vi "系列号查询.vi"() -> ()   [LabVIEW 2016, in "斯坦道多参数.lvlib"]
panel:
  in  "传感器系列号":T1
  in  "布尔":bool
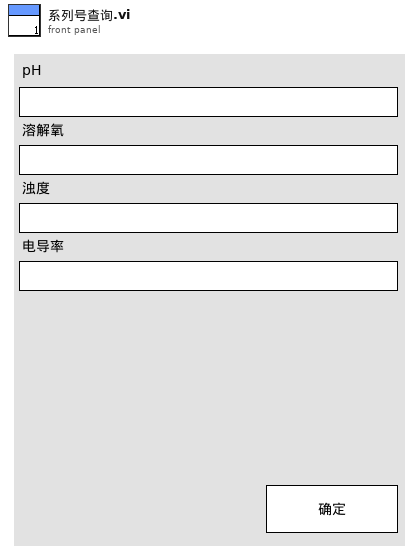
[diagram p1: front panel]
types:
  T1 = cluster{"pH":string, "溶解氧":string, "浊度":string, "电导率":string, "ORP":string, "叶绿素a":string, "藻密度":string}
  T2 = cluster{"pH探头选择":u16, "DO探头选择":u16, "电导率探头选择":u16, "浊度探头选择":u16, "叶绿素a探头选择":u16, "蓝绿藻探头选择":u16, "orp探头选择":u16, "COD探头选择":u16, "DO2探头选择":u16}
  T3 = enum16{"null", "pH", "DO", "浊度", "电导率", "叶绿素a", "DO2"}
  T4 = cluster{"电极状态标志":u16, "电极型号标志":u16, "电导率测量值":sgl, "温度测量值":sgl, "电导率信号值":sgl, "温度信号值":sgl, "温度补偿系数":sgl, "电导率偏移修正值":sgl, "温度偏移修正值":sgl, "手动温度补偿值":sgl, "电导率电极零点":sgl, "电导率电极斜率":sgl, "命令滤波设定":u16, "温度模式":enum16{"ATC", "MTC"}, "生产批次":u16, "电极序号":u16, "串口地址":u16, "串口波特率":enum16{"9600", "19200", "115200"}, "串口校验位":enum16{"NONE", "ODD", "EVEN"}, "串口停止位":enum16{"1bit", "2bit"}, "第一点标准值":sgl, "第二点标准值":sgl}
  T5 = cluster{"报警码":u16, "电导率数据（uS/cm）":sgl, "0x0003 NC":sgl, "温度数据":sgl, "电导率原始信号电阻":sgl, "当前量程":u16, "温度补偿系数":sgl, "0X0009_NC":string, "产品名称":string, "序列号":string, "硬件版本":string, "软件版本":string, "通讯地址":u16, "波特率":u16, "设备类型":u16, "0X0026_NC":string, "第一点原始数据":sgl, "第一点校准数据":sgl, "0X0035_NC":sgl, "0X0037_NC":sgl, "探头校准命令":u16, "温度校准参数":sgl, "温度校准命令":u16}
  T6 = cluster{"报警码":u16, "叶绿素a":sgl, "温度数据":sgl, "原始光强数值":u16, "量程":u16, "平均次数":u16, "清扫模式":u16, "清扫次数":u16, "清扫间隔分钟":u16, "0X000B_NC":string, "产品名称":string, "序列号":string, "硬件版本":string, "软件版本":string, "通讯地址":u16, "波特率":u16, "设备类型":u16, "0X0026_NC":string, "校准量程":u16, "第一点原始光强":u16, "第一点校准数据":sgl, "第二点原始光强":u16, "第二点校准数据":sgl, "第三点原始光强":u16, "第三点校准数据":sgl, "探头校准命令":u16, "温度校准参数":sgl, "温度校准命令":u16}
  T7 = cluster{"电极状态标志":u16, "电极型号标志":u16, "酸碱度测量值":sgl, "温度测量值":sgl, "酸碱度信号值":sgl, "温度信号值":sgl, "酸碱度偏移修正值":sgl, "温度偏移修正值":sgl, "手动温度补偿值":sgl, "酸碱度电极零点":sgl, "酸碱度电极斜率":sgl, "第1点标准值记录":sgl, "第1点信号值记录":sgl, "第1点温度值记录":sgl, "第2点标准值记录":sgl, "第2点信号值记录":sgl, "第2点温度值记录":sgl, "命令滤波设定":u16, "温度模式":enum16{"ATC", "MTC"}, "生产批次":u16, "电极序号":u16, "串口地址":u16, "串口波特率":enum16{"9600", "19200", "115200"}, "串口校验位":enum16{"NONE", "ODD", "EVEN"}, "串口停止位":enum16{"1bit", "2bit"}, "第一点标准值":sgl, "第二点标准值":sgl}
  T8 = cluster{"报警码":u16, "pH数值":sgl, "0X0003_NC":sgl, "温度数据":sgl, "pH原始信号 mv":sgl, "0X0009_NC":string, "产品名称":string, "序列号":string, "硬件版本":string, "软件版本":string, "通讯地址":u16, "波特率":u16, "设备类型":u16, "0X0026_NC":string, "第一点原始数据":sgl, "第一点校准数据":sgl, "第二点原始数据":sgl, "第二点校准数据":sgl, "探头校准命令":u16, "温度校准参数":sgl, "温度校准命令":u16}
  T9 = cluster{"电极状态标志":u16, "电极型号标志":u16, "溶解氧测量值":sgl, "温度测量值":sgl, "溶解氧饱和度值":sgl, "盐度补偿值":sgl, "大气压补偿值":sgl, "溶解氧偏移修正值":sgl, "温度偏移修正值":sgl, "手动温度补偿值":sgl, "溶解氧电极零点":sgl, "溶解氧电极斜率":sgl, "第1点标准值记录":sgl, "第1点信号值记录":sgl, "第1点温度值记录":sgl, "第2点标准值记录":sgl, "第2点信号值记录":sgl, "第2点温度值记录":sgl, "命令滤波设定":u16, "温度模式":enum16{"ATC", "MTC"}, "生产批次":u16, "电极序号":u16, "串口地址":u16, "串口波特率":enum16{"9600", "19200", "115200"}, "串口校验位":enum16{"NONE", "ODD", "EVEN"}, "串口停止位":enum16{"1bit", "2bit"}, "第一点标准值":sgl, "第二点标准值":sgl}
  T10 = cluster{"报警码":u16, "溶解氧数值（mg/L）":sgl, "溶解氧数据（%）":sgl, "温度数据":sgl, "溶解氧原始信号 nA":sgl, "大气压力":sgl, "盐度":sgl, "0X0009_NC":string, "产品名称":string, "序列号":string, "硬件版本":string, "软件版本":string, "通讯地址":u16, "波特率":u16, "设备类型":u16, "0X0026_NC":string, "第一点原始数据":sgl, "第一点校准数据":sgl, "第二点原始数据":sgl, "第二点校准数据":sgl, "探头校准命令":u16, "温度校准参数":sgl, "温度校准命令":u16}
  T11 = cluster{"电极状态标志":u16, "电极型号标志":u16, "浊度测量值":sgl, "温度测量值":sgl, "浊度信号值":sgl, "浊度偏移修正值":sgl, "温度偏移修正值":sgl, "手动温度补偿值":sgl, "浊度电极零点":sgl, "浊度电极斜率":sgl, "清洁周期":u16, "命令滤波设定":u16, "温度模式":enum16{"ATC", "MTC"}, "生产批次":u16, "电极序号":u16, "串口地址":u16, "串口波特率":enum16{"9600", "19200", "115200"}, "串口校验位":enum16{"NONE", "ODD", "EVEN"}, "串口停止位":enum16{"1bit", "2bit"}, "第一点标准值":sgl, "第二点标准值":sgl, "第三点标准值":sgl}
  T12 = cluster{"报警码":u16, "浊度数值 NTU":sgl, "温度数据":sgl, "原始光强数值":u16, "量程":u16, "平均次数":u16, "清扫模式":u16, "清扫次数":u16, "清扫间隔分钟":u16, "0X000B_NC":string, "产品名称":string, "序列号":string, "硬件版本":string, "软件版本":string, "通讯地址":u16, "波特率":u16, "设备类型":u16, "0X0026_NC":string, "校准量程":u16, "第一点原始光强":u16, "第一点校准数据":sgl, "第二点原始光强":u16, "第二点校准数据":sgl, "第三点原始光强":u16, "第三点校准数据":sgl, "探头校准命令":u16, "温度校准参数":sgl, "温度校准命令":u16}
  T13 = cluster{"电极状态标志":u16, "电极型号标志":u16, "测量值":sgl, "温度测量值":sgl, "信号值":sgl, "温度信号值":sgl, "000AH_NC":sgl, "偏移修正值":sgl, "温度偏移修正值":sgl, "手动温度补偿值":sgl, "命令滤波设定":u16, "温度模式":enum16{"ATC", "MTC"}, "生产批次":u16, "传感器序号":u16, "串口地址":u16, "串口波特率":enum16{"9600", "19200", "115200"}, "串口校验位":enum16{"NONE", "ODD", "EVEN"}, "串口停止位":enum16{"1bit", "2bit"}}
  T14 = cluster{"报警码":u16, "蓝绿藻":sgl, "温度数据":sgl, "原始光强数值":u16, "量程":u16, "平均次数":u16, "清扫模式":u16, "清扫次数":u16, "清扫间隔分钟":u16, "0X000B_NC":string, "产品名称":string, "序列号":string, "硬件版本":string, "软件版本":string, "通讯地址":u16, "波特率":u16, "设备类型":u16, "0X0026_NC":string, "校准量程":u16, "第一点原始光强":u16, "第一点校准数据":sgl, "第二点原始光强":u16, "第二点校准数据":sgl, "第三点原始光强":u16, "第三点校准数据":sgl, "探头校准命令":u16, "温度校准参数":sgl, "温度校准命令":u16}
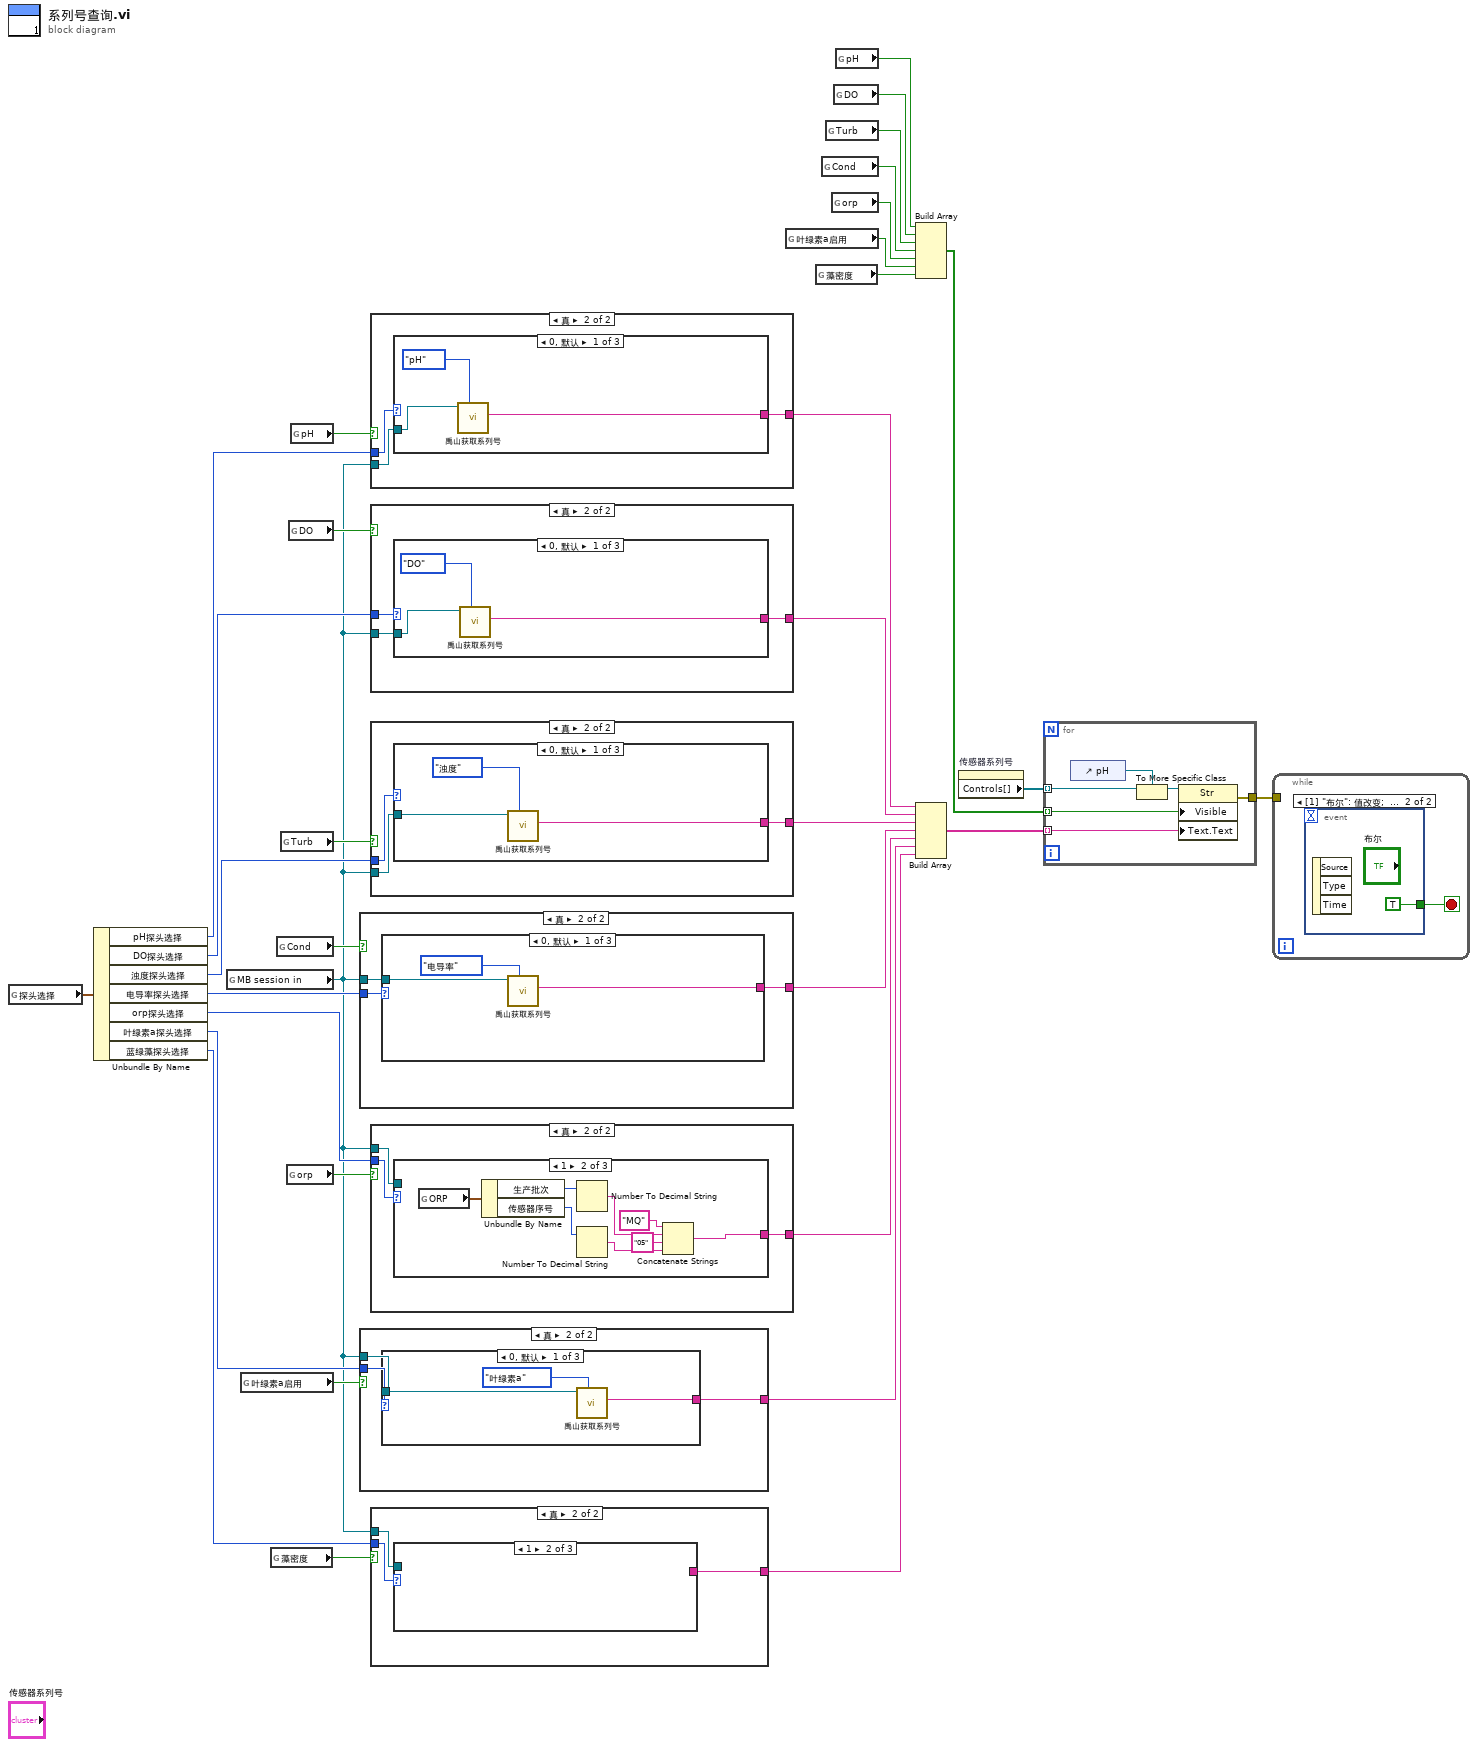
[diagram p0: block diagram]
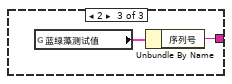
[diagram p4: hidden frame]
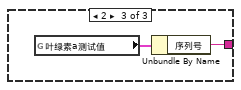
[diagram p7: hidden frame]
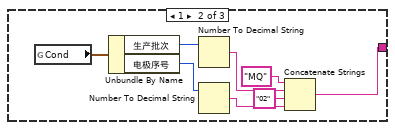
[diagram p12: hidden frame]
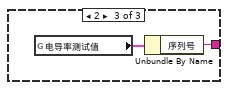
[diagram p13: hidden frame]
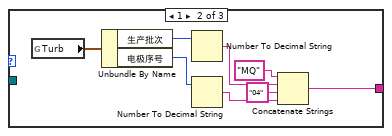
[diagram p15: hidden frame]
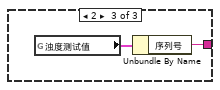
[diagram p16: hidden frame]
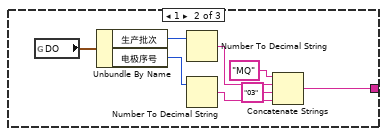
[diagram p18: hidden frame]
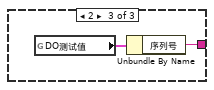
[diagram p19: hidden frame]
diagram:
  n1 = global read "断电保存变量.vi" "探头选择"() -> (w24:T2)
  n2 = Unbundle By Name(w24) -> ("pH探头选择"=w23:u16, "DO探头选择"=w21:u16, "浊度探头选择"=w19:u16, "电导率探头选择"=w16:u16, "orp探头选择"=w15:u16, "叶绿素a探头选择"=w13:u16, "蓝绿藻探头选择"=w9:u16)
  n3 = global read "多参数全局变量.vi" "MB session in"() -> (w10:refnum<class "MB_Master.lvclass">)
  n4 = global read "断电保存变量.vi" "叶绿素a启用"() -> (w12:bool)
  n5 = global read "断电保存变量.vi" "藻密度"() -> (w11:bool)
  n6 = global read "断电保存变量.vi" "Cond"() -> (w17:bool)
  n7 = global read "断电保存变量.vi" "Turb"() -> (w18:bool)
  n8 = global read "断电保存变量.vi" "orp"() -> (w14:bool)
  n9 = global read "断电保存变量.vi" "DO"() -> (w20:bool)
  n10 = global read "断电保存变量.vi" "pH"() -> (w22:bool)
  n11 = case shown="真" w17 {
    tunnel: w16 -> [_ w37]
    tunnel: [_ w36] -> w5
    tunnel: w10 -> [_ w35]
    frame False {
    }
    frame True {
      n12 = case shown="0, 默认" w37 {
        tunnel: w35 -> [w40 _ _]
        tunnel: [w39 w44 w49] -> w36
        frame 0, Default {
          n13 = call "禹山获取系列号.vi"("探头"=T3."电导率", "MB session in"=w40) -> ("SN"=w39:string)  [unwired: 7 in, 2 out]
        }
        frame 1 {
          n14 = global read "国弘过程全局变量.vi" "Cond"() -> (w45:T4)
          n15 = Unbundle By Name(w45) -> ("生产批次"=w46:u16, "电极序号"=w47:u16)
          n16 = Number To Decimal String(number=w46) -> (decimal integer string=w48:string)  [unwired: 1 in]
          n17 = Number To Decimal String(number=w47) -> (decimal integer string=w42:string)  [unwired: 1 in]
          n18 = Concatenate Strings("MQ" ("字符串"), w48, "02" ("字符串"), w42) -> (w44:string)
        }
        frame 2 {
          n19 = global read "纳清过程全局变量.vi" "电导率测试值"() -> (w50:T5)
          n20 = Unbundle By Name(w50) -> ("序列号"=w49:string)
        }
      }
    }
  }
  n21 = case shown="真" w12 {
    tunnel: w13 -> [_ w53]
    tunnel: [_ w52] -> w3
    tunnel: w10 -> [_ w51]
    frame False {
    }
    frame True {
      n22 = case shown="0, 默认" w53 {
        tunnel: w51 -> [w56 _ _]
        tunnel: [w55 _ w57] -> w52
        frame 0, Default {
          n23 = call "禹山获取系列号.vi"("探头"=T3."叶绿素a", "MB session in"=w56) -> ("SN"=w55:string)  [unwired: 7 in, 2 out]
        }
        frame 1 {
        }
        frame 2 {
          n24 = global read "纳清过程全局变量.vi" "叶绿素a测试值"() -> (w58:T6)
          n25 = Unbundle By Name(w58) -> ("序列号"=w57:string)
        }
      }
    }
  }
  n26 = case shown="真" w22 {
    tunnel: w23 -> [_ w61]
    tunnel: [_ w60] -> w8
    tunnel: w10 -> [_ w59]
    frame False {
    }
    frame True {
      n27 = case shown="0, 默认" w61 {
        tunnel: w59 -> [w64 _ _]
        tunnel: [w63 w68 w73] -> w60
        frame 0, Default {
          n28 = call "禹山获取系列号.vi"("探头"=T3."pH", "MB session in"=w64) -> ("SN"=w63:string)  [unwired: 7 in, 2 out]
        }
        frame 1 {
          n29 = global read "国弘过程全局变量.vi" "pH"() -> (w69:T7)
          n30 = Unbundle By Name(w69) -> ("生产批次"=w70:u16, "电极序号"=w71:u16)
          n31 = Number To Decimal String(number=w70) -> (decimal integer string=w72:string)  [unwired: 1 in]
          n32 = Number To Decimal String(number=w71) -> (decimal integer string=w66:string)  [unwired: 1 in]
          n33 = Concatenate Strings("MQ" ("字符串"), w72, "01" ("字符串"), w66) -> (w68:string)
        }
        frame 2 {
          n34 = global read "纳清过程全局变量.vi" "pH测试值"() -> (w74:T8)
          n35 = Unbundle By Name(w74) -> ("序列号"=w73:string)
        }
      }
    }
  }
  n36 = case shown="真" w20 {
    tunnel: w21 -> [_ w77]
    tunnel: [_ w76] -> w7
    tunnel: w10 -> [_ w75]
    frame False {
    }
    frame True {
      n37 = case shown="0, 默认" w77 {
        tunnel: w75 -> [w80 _ _]
        tunnel: [w79 w84 w89] -> w76
        frame 0, Default {
          n38 = call "禹山获取系列号.vi"("探头"=T3."DO", "MB session in"=w80) -> ("SN"=w79:string)  [unwired: 7 in, 2 out]
        }
        frame 1 {
          n39 = global read "国弘过程全局变量.vi" "DO"() -> (w85:T9)
          n40 = Unbundle By Name(w85) -> ("生产批次"=w86:u16, "电极序号"=w87:u16)
          n41 = Number To Decimal String(number=w86) -> (decimal integer string=w88:string)  [unwired: 1 in]
          n42 = Number To Decimal String(number=w87) -> (decimal integer string=w82:string)  [unwired: 1 in]
          n43 = Concatenate Strings("MQ" ("字符串"), w88, "03" ("字符串"), w82) -> (w84:string)
        }
        frame 2 {
          n44 = global read "纳清过程全局变量.vi" "DO测试值"() -> (w90:T10)
          n45 = Unbundle By Name(w90) -> ("序列号"=w89:string)
        }
      }
    }
  }
  n46 = case shown="真" w18 {
    tunnel: w19 -> [_ w93]
    tunnel: [_ w92] -> w6
    tunnel: w10 -> [_ w91]
    frame False {
    }
    frame True {
      n47 = case shown="0, 默认" w93 {
        tunnel: w91 -> [w96 _ _]
        tunnel: [w95 w100 w105] -> w92
        frame 0, Default {
          n48 = call "禹山获取系列号.vi"("探头"=T3."浊度", "MB session in"=w96) -> ("SN"=w95:string)  [unwired: 7 in, 2 out]
        }
        frame 1 {
          n49 = global read "国弘过程全局变量.vi" "Turb"() -> (w101:T11)
          n50 = Unbundle By Name(w101) -> ("生产批次"=w102:u16, "电极序号"=w103:u16)
          n51 = Number To Decimal String(number=w102) -> (decimal integer string=w104:string)  [unwired: 1 in]
          n52 = Number To Decimal String(number=w103) -> (decimal integer string=w98:string)  [unwired: 1 in]
          n53 = Concatenate Strings("MQ" ("字符串"), w104, "04" ("字符串"), w98) -> (w100:string)
        }
        frame 2 {
          n54 = global read "纳清过程全局变量.vi" "浊度测试值"() -> (w106:T12)
          n55 = Unbundle By Name(w106) -> ("序列号"=w105:string)
        }
      }
    }
  }
  n56 = case shown="真" w14 {
    tunnel: w15 -> [_ w109]
    tunnel: [_ w108] -> w4
    tunnel: w10 -> [_ w107]
    frame False {
    }
    frame True {
      n57 = case shown="1" w109 {
        tunnel: w107 -> [_ _ _]
        tunnel: [_ w113 _] -> w108
        frame 0, Default {
        }
        frame 1 {
          n58 = global read "国弘过程全局变量.vi" "ORP"() -> (w114:T13)
          n59 = Unbundle By Name(w114) -> ("生产批次"=w115:u16, "传感器序号"=w116:u16)
          n60 = Number To Decimal String(number=w115) -> (decimal integer string=w117:string)  [unwired: 1 in]
          n61 = Number To Decimal String(number=w116) -> (decimal integer string=w111:string)  [unwired: 1 in]
          n62 = Concatenate Strings("MQ" ("字符串"), w117, "05" ("字符串"), w111) -> (w113:string)
        }
        frame 2 {
        }
      }
    }
  }
  n63 = case shown="真" w11 {
    tunnel: w9 -> [_ w120]
    tunnel: [_ w119] -> w2
    tunnel: w10 -> [_ w118]
    frame False {
    }
    frame True {
      n64 = case shown="1" w120 {
        tunnel: w118 -> [_ _ _]
        tunnel: [_ _ w121] -> w119
        frame 0, Default {
        }
        frame 1 {
        }
        frame 2 {
          n65 = global read "纳清过程全局变量.vi" "蓝绿藻测试值"() -> (w122:T14)
          n66 = Unbundle By Name(w122) -> ("序列号"=w121:string)
        }
      }
    }
  }
  n67 = global read "断电保存变量.vi" "叶绿素a启用"() -> (w29:bool)
  n68 = global read "断电保存变量.vi" "藻密度"() -> (w28:bool)
  n69 = global read "断电保存变量.vi" "Cond"() -> (w31:bool)
  n70 = global read "断电保存变量.vi" "Turb"() -> (w32:bool)
  n71 = global read "断电保存变量.vi" "orp"() -> (w30:bool)
  n72 = global read "断电保存变量.vi" "DO"() -> (w33:bool)
  n73 = global read "断电保存变量.vi" "pH"() -> (w34:bool)
  n74 = Build Array(w34, w33, w32, w31, w30, w29, w28) -> (w26:bool[])
  n75 = Build Array(w8, w7, w6, w5, w4, w3, w2) -> (w1:string[])
  n76 = property on="传感器系列号" class="Clust (严格)"() -> ("Controls[]"=w27:refnum<vi>[])  [unwired: 2 in, 2 out]
  n77 = for {
    tunnel: w27 -> [w126] mode=indexing
    tunnel: w26 -> [w128] mode=indexing
    tunnel: [w127] -> w25
    tunnel: w1 -> [w123] mode=indexing
    n78 = control-ref of="pH"() -> (w125:refnum<vi>)
    n79 = To More Specific Class(target class=w125, reference=w126) -> (specific class reference=w124:refnum<vi>)  [unwired: 1 in, 1 out]
    n80 = property class="Str"(reference=w124, "Visible"=w128, "Text.Text"=w123) -> (error out=w127:errorcluster)  [unwired: 1 in, 1 out]
  }
  n81 = while {
    tunnel: w25 -> [_]
    stop <- w129 stop-if-true
    n82 = event shown="[1] \"布尔\": 值改变;  前面板关闭" {
      selector: _ -> [_ _]
      dyn-events: _ -> [_ _]
      timeout: _ -> [_ _]
      tunnel: [_ TRUE] -> w129
      event Timeout {
        n83 = event-data() -> ()  [unwired: 1 in, 3 out]
      }
      event "布尔": Value Change; Panel Close {
        n84 = event-data() -> ()  [unwired: 1 in, 3 out]
      }
    }
  }
